vi "Water Control Normally Closed.vi"(11 "Cooling Water Control Valve (% Open)":dbl) -> (3 "Array":dbl[](array[numeric]))   [LabVIEW 2017]
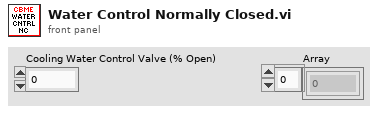
[diagram p1: front panel]
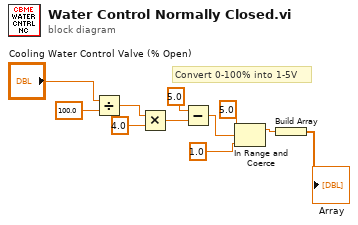
[diagram p0: block diagram]
diagram:
  # "Convert 0-100% into 1-5V"
  n1 = Divide(x="Cooling Water Control Valve (% Open)", y=100.0) -> (x/y=w3:dbl)
  n2 = Multiply(x=w3, y=4.0) -> (x*y=w5:dbl)
  n3 = Subtract(x=5.0 ("y"), y=w5) -> (x-y=w7:dbl)
  n4 = In Range and Coerce(upper limit=5.0, x=w7, lower limit=1.0) -> (coerced(x)=w11:dbl)  [unwired: 1 out]
  n5 = Build Array(w11) -> (→"Array":dbl[])
